vi "svx_SC Line Manage Grid.vi"(4 "Minor Color":u32, 5 "enable update?":bool=TRUE, 6 "Major Color":u32, 7 "Axis":enum16{"X-Scale", "Y-Scale", "Z-Scale"}(ring), 10 "Grid Style":u16, 11 "Shaft Centerline in":refnum<vi>) -> (0 "actual minor":u32, 1 "actual major":u32, 3 "Shaft Centerline out":refnum<vi>)   [LabVIEW 2017, in "SVX SC Line.xctl"]
uses:
  <vilib>/addons/_XControls/Shaft Centerline/SVX SC Line.xctl
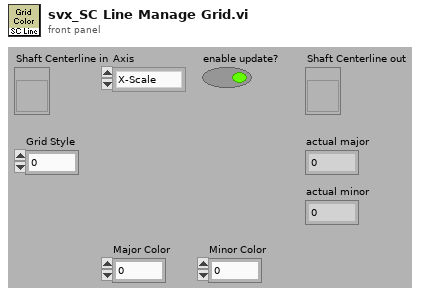
[diagram p1: front panel]
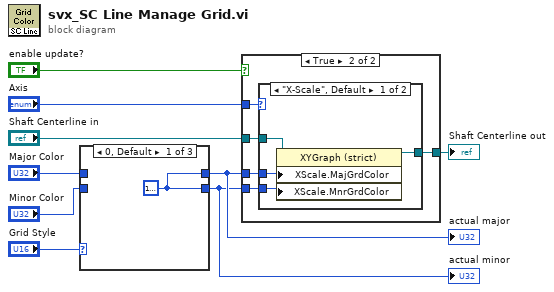
[diagram p0: block diagram]
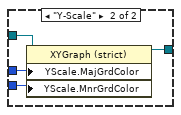
[diagram p3: hidden frame]
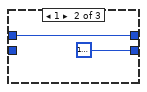
[diagram p4: hidden frame]
diagram:
  n1 = case shown="0, Default" "Grid Style" {
    tunnel: [w10 w11 w14] -> w9
    tunnel: [w10 u32 16777216 w13] -> w7
    tunnel: "Major Color" -> [_ w11 w14]
    tunnel: "Minor Color" -> [_ _ w13]
    frame 0, Default {
      w10 = u32 16777216
    }
    frame 1 {
    }
    frame 2 {
    }
  }
  "actual major" <- w9
  "actual minor" <- w7
  n2 = case shown="True" "enable update?" {
    tunnel: w9 -> [_ w20]
    tunnel: w7 -> [_ w19]
    tunnel: "Axis" -> [_ w18]
    tunnel: "Shaft Centerline in" -> [w15 w17]
    tunnel: [w15 w16] -> w2
    frame False {
    }
    frame True {
      n3 = case shown="\"X-Scale\", Default" w18 {
        tunnel: w20 -> [w24 w28]
        tunnel: w17 -> [w23 w27]
        tunnel: w19 -> [w22 w26]
        tunnel: [w21 w25] -> w16
        frame "X-Scale", Default {
          n4 = property class="XYGraph (strict)"(reference=w23, "XScale.MajGrdColor"=w24, "XScale.MnrGrdColor"=w22) -> (reference out=w21:refnum<vi>)  [unwired: 1 in, 1 out]
        }
        frame "Y-Scale" {
          n5 = property class="XYGraph (strict)"(reference=w27, "YScale.MajGrdColor"=w28, "YScale.MnrGrdColor"=w26) -> (reference out=w25:refnum<vi>)  [unwired: 1 in, 1 out]
        }
      }
    }
  }
  "Shaft Centerline out" <- w2
